vi "Buffered Log Sink Example.vi"() -> ()   [LabVIEW 2019, in "Logger Examples.lvlib"]
uses:
  <vilib>/gpm_packages/@cs/event-logger/Examples/Logger Examples.lvlib
  <vilib>/gpm_packages/@cs/event-logger/Source/Composed Log/Types/Log Level.ctl
  <vilib>/gpm_packages/@cs/event-logger/Source/String Formats/String Expression Format/String Expression Format.lvclass/String Expression Format.ctl
  <vilib>/gpm_packages/@cs/event-logger/Source/Composed Log/LoggerReference/LoggerReference.lvclass/LoggerReference.ctl
  601d143e-8928-4a3b-9174-3083e729aaa9.vi
  <vilib>/gpm_packages/@cs/event-logger/Source/String Formats/String Expression Format/Run Formatter.vi
  <vilib>/gpm_packages/@cs/event-logger/Source/Composed Log/LoggerReference/Return Aggregate Queues.vi
  <vilib>/gpm_packages/@cs/event-logger/Source/Composed Log/LoggerReference/Add Aggregate Log.vi
  601d143e-8928-4a3b-9174-3083e729aaa9.vi/a3da3afa-ac43-4bb3-81ff-a2729e80cca6.vi
  <vilib>/gpm_packages/@cs/event-logger/Source/Composed Log/LoggerReference/Log.vi
  <vilib>/gpm_packages/@cs/event-logger/Source/Composed Log/LoggerReference/Get Valid Event Time.vi
  <vilib>/dlg_ctls.llb/Space Constant.vi
  <vilib>/gpm_packages/@cs/event-logger/Source/Composed Log/LoggerReference/Send Add Sink.vi
  <vilib>/gpm_packages/@cs/event-logger/Source/Composed Log/LoggerReference/Remove Stale Logs.vi
  <vilib>/gpm_packages/@cs/event-logger/Source/String Formats/String Expression Format/String Expression Format.lvclass
  C:/Program Files/National Instruments/LabVIEW 2019/vi.lib/gpm_packages/@cs/event-logger/Source/IStringFormat/IStringFormat.lvclass
  <vilib>/gpm_packages/@cs/event-logger/Source/String Control Sink/String Control Sink.lvclass
  C:/Program Files/National Instruments/LabVIEW 2019/vi.lib/gpm_packages/@cs/event-logger/Source/Composed Log/Log Sink/Log Sink.lvclass
  <vilib>/gpm_packages/@cs/event-logger/Source/Buffered Log Sink/Buffered Log Sink.lvclass
  <vilib>/gpm_packages/@cs/event-logger/Source/Composed Log/Application Logger/Launch Worker Loop.vi
  <vilib>/gpm_packages/@cs/event-logger/Source/Composed Log/LoggerReference/Initialize Logger Instance.vi
  <vilib>/gpm_packages/@cs/event-logger/Source/Composed Log/LoggerReference/LoggerReference.lvclass
  <vilib>/gpm_packages/@cs/event-logger/Source/Composed Log/IErrorFormat/IErrorFormat.lvclass
  <vilib>/gpm_packages/@cs/event-logger/Source/Composed Log/Log Sink/Log Sink.lvclass
  <vilib>/gpm_packages/@cs/event-logger/Source/Composed Log/Composed Log.lvlib
panel:
  in  "Log Error":bool
  in  "Error Information":string
  in  "Error Code":i32
  in  "Event Level":T1(ring)
  out "1S Timeout, 5 Element Buffer":string
  out "No Timeout - 5 Element Buffer":string
  out "500mS Timeout, Unlimited Buffer":string
  in  "Data To Log":string
  in  "Source":string="User"
  in  "Log":bool
  # "This Sink will only log events once its buffer is full. Any unlogged events will be logged on shutdown."
  # "This Sink will only log events once its timer elapses. Any unlogged events will be logged on shutdown."
  # "This Sink will log events when its buffer is full, or its timer elapses. Any unlogged events will be logged on shutdown."
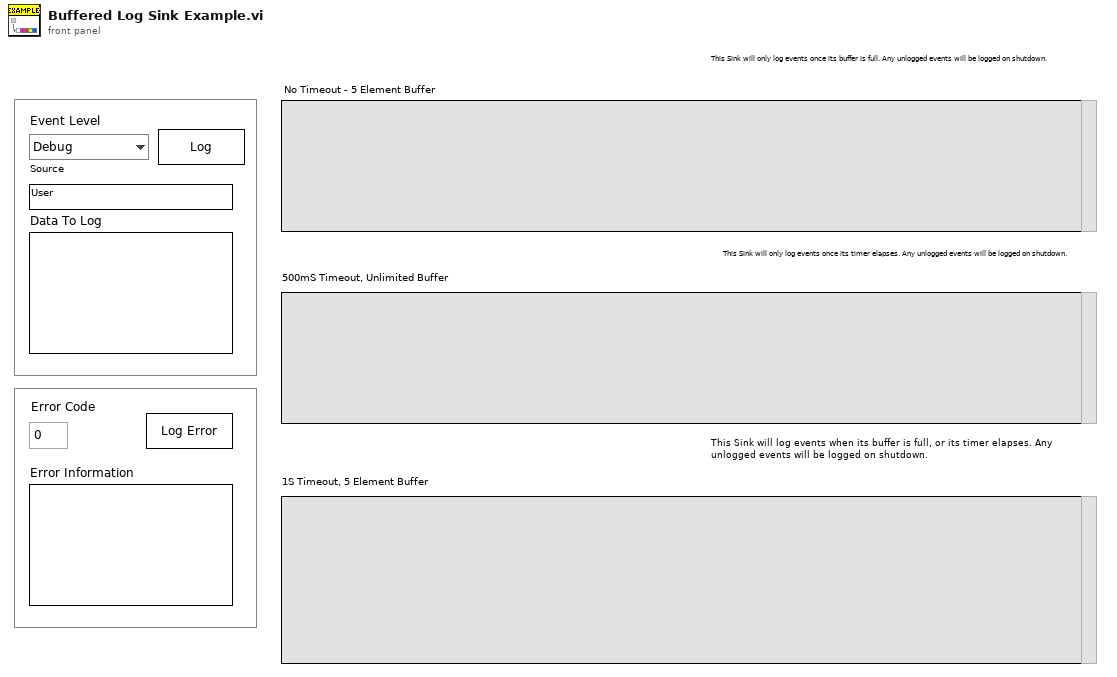
[diagram p1: front panel]
types:
  T1 = enum16{"Debug", "Info", "Warning", "Error", "Critical"}
  T2 = typedef "Composed Log.lvlib/Log Level.ctl" = enum16{"Debug", "Info", "Warning", "Error", "Critical"}
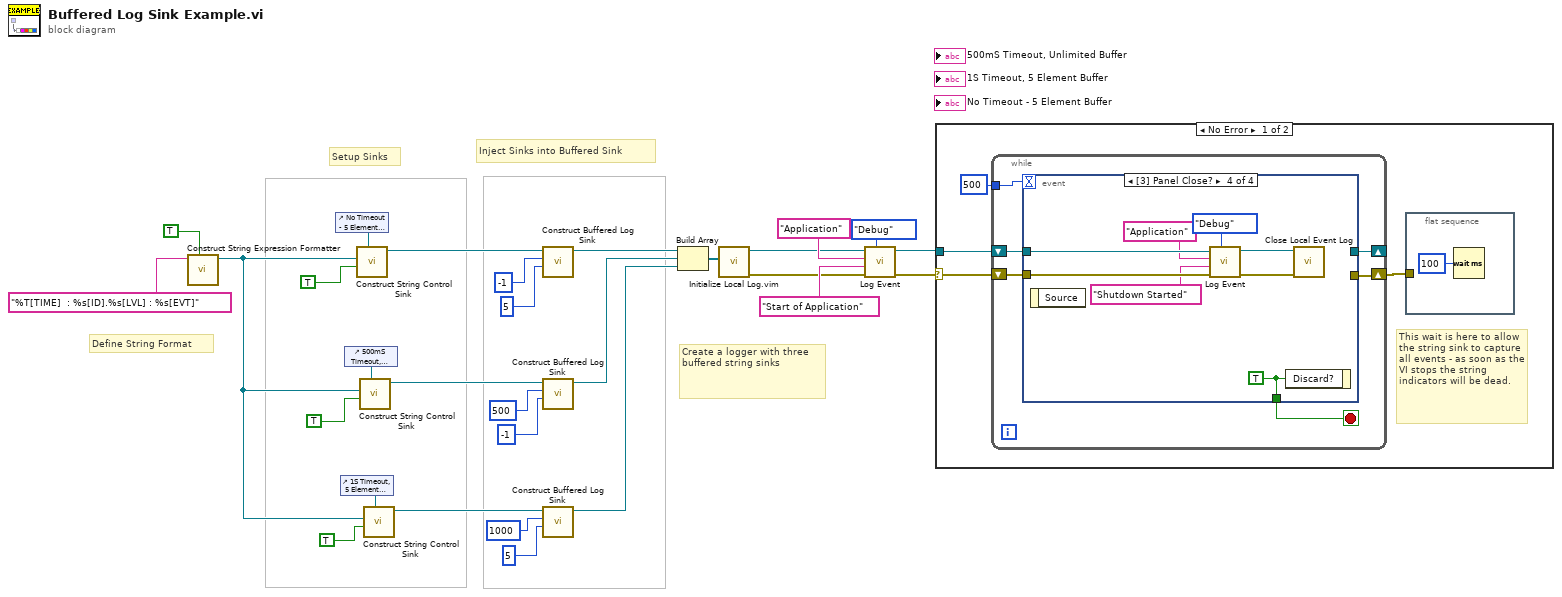
[diagram p0: block diagram]
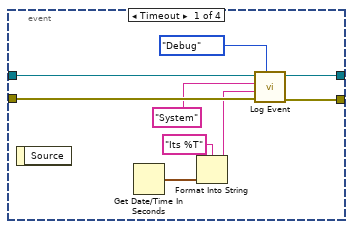
[diagram p2: hidden frame]
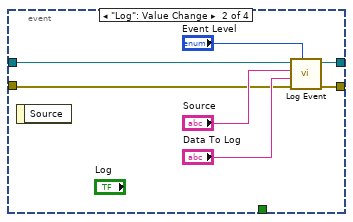
[diagram p3: hidden frame]
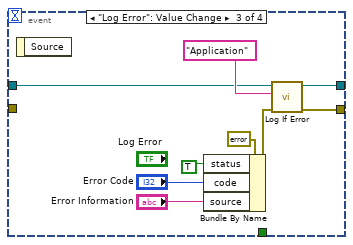
[diagram p4: hidden frame]
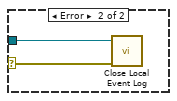
[diagram p5: hidden frame]
diagram:
  # "Inject Sinks into Buffered Sink"
  # "Setup Sinks"
  # "Define String Format"
  # "Create a logger with three buffered string sinks"
  n1 = call <vilib>:"Construct String Expression Formatter.vi"("Append EOL?"=TRUE, "Format Specifier"="%T[TIME]  : %s[ID].%s[LVL] : %s[EVT]") -> ("String Expression Format out"=w2:refnum<class "String Expression Format.lvclass">)  [unwired: 8 in, 1 out]
  n2 = control-ref of="No Timeout - 5 Element Buffer"() -> (w27:refnum<vi>)
  n3 = control-ref of="1S Timeout, 5 Element Buffer"() -> (w24:refnum<vi>)
  n4 = control-ref of="500mS Timeout, Unlimited Buffer"() -> (w28:refnum<vi>)
  n5 = call <vilib>:"Construct String Control Sink.vi"("Str Refnum"=w27, "AutoScroll?(F)"=TRUE, "LogFormat"=w2) -> ("String Control Sink out"=w1:refnum<class "String Control Sink.lvclass">)  [unwired: 8 in]
  n6 = call <vilib>:"Construct String Control Sink.vi"("Str Refnum"=w28, "AutoScroll?(F)"=TRUE, "LogFormat"=w2) -> ("String Control Sink out"=w10:refnum<class "String Control Sink.lvclass">)  [unwired: 8 in]
  n7 = call <vilib>:"Construct String Control Sink.vi"("Str Refnum"=w24, "AutoScroll?(F)"=TRUE, "LogFormat"=w2) -> ("String Control Sink out"=w6:refnum<class "String Control Sink.lvclass">)  [unwired: 8 in]
  n8 = call <vilib>:"Construct Buffered Log Sink.vi"("Buffer Size (128)"=5, "Buffer Timeout ms (-1)"=-1, "Sink to Buffer"=w1) -> ("Buffered Log Sink out"=w13:refnum<class "Buffered Log Sink.lvclass">)  [unwired: 8 in]
  n9 = call <vilib>:"Construct Buffered Log Sink.vi"("Buffer Size (128)"=-1, "Buffer Timeout ms (-1)"=500, "Sink to Buffer"=w10) -> ("Buffered Log Sink out"=w9:refnum<class "Buffered Log Sink.lvclass">)  [unwired: 8 in]
  n10 = call <vilib>:"Construct Buffered Log Sink.vi"("Buffer Size (128)"=5, "Buffer Timeout ms (-1)"=1000, "Sink to Buffer"=w6) -> ("Buffered Log Sink out"=w5:refnum<class "Buffered Log Sink.lvclass">)  [unwired: 8 in]
  n11 = Build Array(w13, w9, w5) -> (w14:refnum<class "Buffered Log Sink.lvclass">[])
  n12 = call "Initialize Local Log.vim"("Startup Sink(s)"=w14) -> ("error out"=w20:errorcluster, "Log Instance Reference"=w19:refnum<class "LoggerReference.lvclass">)  [unwired: 8 in, 1 out]
  n13 = call <vilib>:"Log Event.vi"("Event Level"=Log_Level."Debug", "error in (no error)"=w20, "Data To Log"="Start of Application", "SourceID"="Application", "Log Instance"=w19) -> ("error out"=w18:errorcluster, "Log Instance Out"=w17:refnum<class "LoggerReference.lvclass">)  [unwired: 5 in]
  n14 = case shown="No Error" w18 {
    selector: w18 -> [w32 w74]
    tunnel: w17 -> [w33 w75]
    frame No Error {
      # "This wait is here to allow the string sink to capture all events - as soon as the VI stops the string indicators will be dead."
      n15 = while {
        shift-right: [w38] -> _
        shift-left: w33 -> [w39]
        shift-right: [w36] -> w30
        shift-left: w32 -> [w37]
        tunnel: 500 -> [w35]
        stop <- w40 stop-if-true
        n16 = event shown="[3] Panel Close?" {
          selector: _ -> [_ _ _ _]
          dyn-events: _ -> [_ _ _ _]
          timeout: w35 -> [_ _ _ _]
          tunnel: [_ _ _ w73] -> w40
          tunnel: w39 -> [w49 w53 w59 w71]
          tunnel: [w48 w51 w57 _] -> w38
          tunnel: w37 -> [w46 w50 _ w72]
          tunnel: [w45 w52 w58 _] -> w36
          event Timeout {
            n17 = event-data() -> ()  [unwired: 1 in, 1 out]
            n18 = Get Date/Time In Seconds() -> (seconds since 1Jan1904=w43:timestamp)
            n19 = Format Into String(format string="Its %T" ("Log Message"), w43) -> (resulting string=w41:string)  [unwired: 2 in, 1 out]
            n20 = call <vilib>:"Log Event.vi"("Event Level"=Log_Level."Debug", "error in (no error)"=w46, "Data To Log"=w41, "SourceID"="System" ("Event Source"), "Log Instance"=w49) -> ("error out"=w45:errorcluster, "Log Instance Out"=w48:refnum<class "LoggerReference.lvclass">)  [unwired: 5 in]
          }
          event "Log": Value Change {
            n21 = event-data() -> ()  [unwired: 1 in, 1 out]
            n22 = call <vilib>:"Log Event.vi"("Event Level"="Event Level", "error in (no error)"=w50, "Data To Log"="Data To Log", "SourceID"="Source", "Log Instance"=w53) -> ("error out"=w52:errorcluster, "Log Instance Out"=w51:refnum<class "LoggerReference.lvclass">)  [unwired: 5 in]
          }
          event "Log Error": Value Change {
            n23 = event-data() -> ()  [unwired: 1 in, 1 out]
            n24 = Bundle By Name(cluster=errorcluster {"status"=FALSE, "code"=0, "source"=""} ("Error In"), "status"=TRUE, "code"="Error Code", "source"="Error Information") -> (w63:errorcluster)
            n25 = call <vilib>:"Log If Error.vi"("Error In"=w63, "SourceID"="Application" ("Source"), "Log Instance"=w59) -> ("error out"=w58:errorcluster, "Log Instance Out"=w57:refnum<class "LoggerReference.lvclass">)  [unwired: 7 in]
          }
          event Panel Close? {
            w73 = TRUE ("Discard?")
            n26 = event-data() -> ()  [unwired: 1 in, 1 out]
            n27 = call <vilib>:"Log Event.vi"("Event Level"=Log_Level."Debug", "error in (no error)"=w72, "Data To Log"="Shutdown Started", "SourceID"="Application", "Log Instance"=w71) -> ("error out"=w70:errorcluster, "Log Instance Out"=w69:refnum<class "LoggerReference.lvclass">)  [unwired: 5 in]
            n28 = event-data("Discard?"=w73) -> ()  [unwired: 1 in, 1 out]
            n29 = call <vilib>:"Close Local Event Log.vi"("error in (no error)"=w70, "Log Instance"=w69) -> ()  [unwired: 9 in, 1 out]
          }
        }
      }
      n30 = flat-sequence {
        tunnel: w30 -> [_]
        frame #0 {
          n31 = Wait (ms)(milliseconds to wait=u32 100) -> ()  [unwired: 1 out]
        }
      }
    }
    frame Error {
      n32 = call <vilib>:"Close Local Event Log.vi"("error in (no error)"=w74, "Log Instance"=w75) -> ()  [unwired: 9 in, 1 out]
    }
  }
